vi "set_written_to_devices.vi"(8 "error in (no error)":errorcluster, 10 "written to devices?":bool[](array[boolean]), 11 "DAQmxWriteSignals in":refnum<class "SignalWriterMM140725DAQmx.lvclass">) -> (0 "error out":errorcluster, 3 "DAQmxWriteSignals out":refnum<class "SignalWriterMM140725DAQmx.lvclass">)   [LabVIEW 2010, in "SignalWriterMM140725DAQmx.lvclass"]
uses:
  SignalWriterMM140725DAQmx.lvclass
  class_data.vi
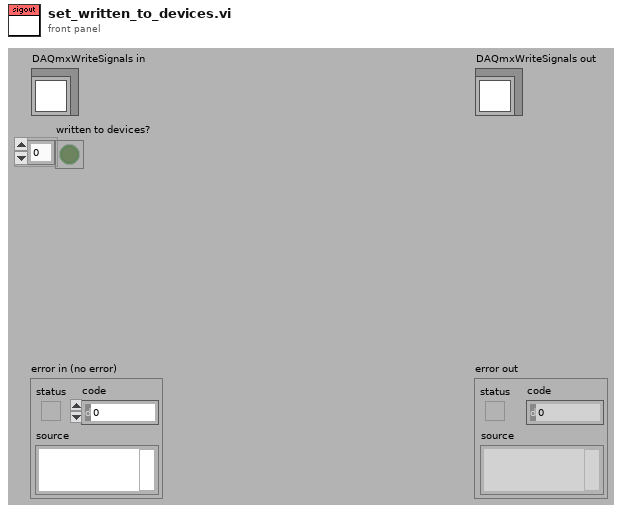
[diagram p1: front panel]
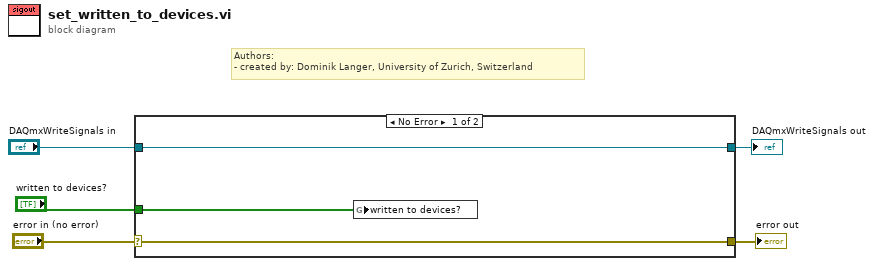
[diagram p0: block diagram]
diagram:
  # "Authors: \n- created by: Dominik Langer, University of Zurich, Switzerland"
  n1 = case shown="No Error" "error in (no error)" {
    selector: "error in (no error)" -> [w7 w10]
    tunnel: [w7 w10] -> w4
    tunnel: [w8 w9] -> w2
    tunnel: "DAQmxWriteSignals in" -> [w8 w9]
    tunnel: "written to devices?" -> [w6 _]
    frame No Error {
      n2 = global write "class_data.vi" "written to devices?"(w6) -> ()
    }
    frame Error {
    }
  }
  "error out" <- w4
  "DAQmxWriteSignals out" <- w2
